vi "Get Measurement.vi"(8 "error in (no error)":errorcluster, 10 "Measurement":T1, 11 "Yokogawa AQ6370D in":refnum<class "Yokogawa AQ6370D.lvclass">) -> (0 "error out":errorcluster, 2 "Measurement Data":dbl, 3 "Yokogawa AQ6370D out":refnum<class "Yokogawa AQ6370D.lvclass">)   [LabVIEW 2018, in "Yokogawa AQ6370D.lvlib" / "Yokogawa AQ6370D.lvclass"]
uses:
  Yokogawa AQ6370D.lvclass
  PPLs/Optical Spectrum Analyzer/Parent/OSA.lvlibp/Custom Controls/enm_Measurement.ctl
  PPLs/Optical Spectrum Analyzer/Parent/OSA.lvlibp/Optical Spectrum Analyzer.lvclass
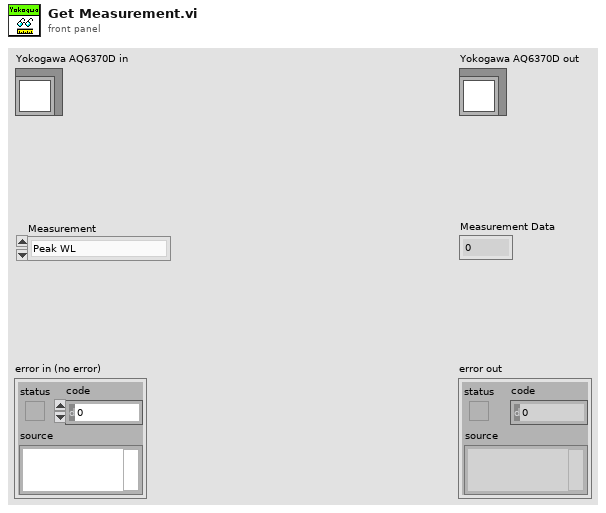
[diagram p1: front panel]
types:
  T1 = typedef "OSA.lvlibp/Optical Spectrum Analyzer.lvclass/enm_Measurement.ctl" = enum16{"Peak WL", "SMSR", "OSNR", "Center WL", "Int. Pwr Spect. Density", "Peak Level", "RMS"}
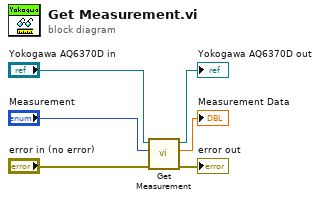
[diagram p0: block diagram]
diagram:
  n1 = call-parent "Get Measurement.vi"("error in (no error)"="error in (no error)", "Measurement"="Measurement", "Optical Spectrum Analyzer in"="Yokogawa AQ6370D in") -> ("error out"=→"error out":errorcluster, "Measurement Data"=→"Measurement Data":dbl, "Optical Spectrum Analyzer out"=→"Yokogawa AQ6370D out":refnum<class "Yokogawa AQ6370D.lvclass">)  [unwired: 6 in]
